vi "xmlparser.vi"(10 "xml_file_content":string="<?xml version=\"1.0\" ?>\n<SC0>\n  <mod0>\n    <ai1>\n      <Cluster>\n        <Name></Name>\n        <NumElts>7</NumElts>\n        <DBL>\n          <Name>max</Name>\n          <Val>10</Val>\n        </DBL>\n        <DBL>\n          <Name>min</Name>\n          <Val>-10</Val>\n        </DBL>\n        <DBL>\n          <Name>factor_a</Name>\n          <Val>22.4</Val>\n        </DBL>\n        <DBL>\n          <Name>factor_b</Name>\n          <Val>0.0</Val>\n        </DBL>\n        <Boolean>\n          <Name>lowpass</Name>\n          <Val>1</Val>\n        </Boolean>\n        <DBL>\n          <Name>lowpassfreq</Name>\n          <Val>60</Val>\n        </DBL>\n        <DBL>\n          <Name>excitation</Name>\n          <Val>0.4</Val>\n        </DBL>\n      </Cluster>\n      <type>VoltageInputExtExc</type>\n      <name>234</name>\n    </ai1>\n    <ai0>\n      <Cluster>\n        <Name></Name>\n        <NumElts>7</NumElts>\n        <DBL>\n          <Name>max</Name>\n          <Val>10</Val>\n        </DBL>\n        <DBL>\n          <Name>min</Name>\n          <Val>-10</Val>\n        </DBL>\n        <DBL>\n          <Name>factor_a</Name>\n          <Val>22.4</Val>\n        </DBL>\n        <DBL>\n          <Name>factor_b</Name>\n          <Val>0.0</Val>\n        </DBL>\n        <Boolean>\n          <Name>lowpass</Name>\n          <Val>1</Val>\n        </Boolean>\n        <DBL>\n          <Name>lowpassfreq</Name>\n          <Val>60</Val>\n        </DBL>\n        <DBL>\n          <Name>excitation</Name>\n          <Val>10</Val>\n        </DBL>\n      </Cluster>\n      <type>VoltageInputIntExc</type>\n      <name>234</name>\n    </ai0>\n  </mod0>\n</SC0>\n", 11 "XPath expression":string) -> (3 "Array 2":string[](array[string]))   [LabVIEW 2011]
uses:
  <vilib>/xml/Close Reference(Node).vi
  <vilib>/xml/NI_XML.lvlib
  Program Files (x86)/National Instruments/LabVIEW 2011/resource/objmgr/DOMUserDefRef.rc
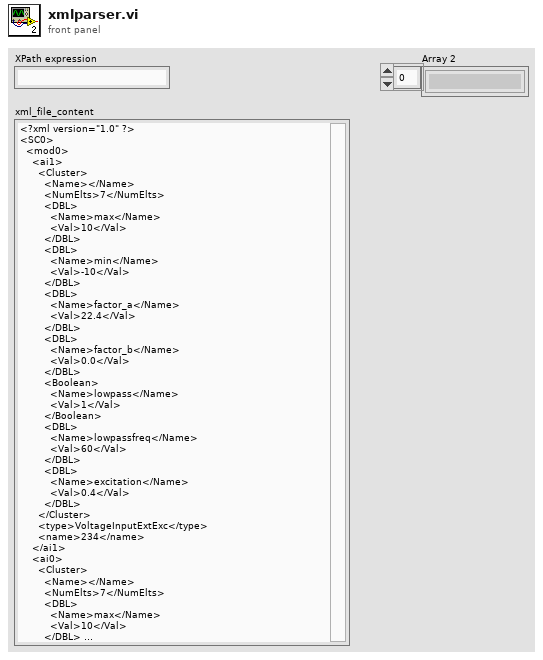
[diagram p1: front panel]
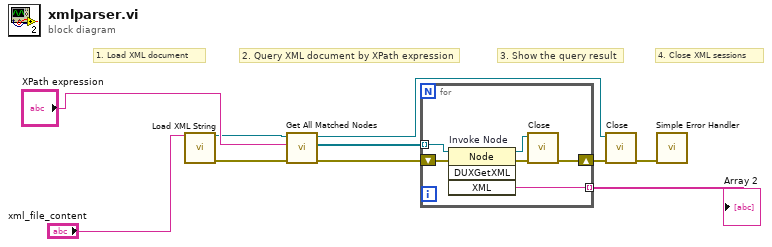
[diagram p0: block diagram]
diagram:
  # "4. Close XML sessions"
  # "3. Show the query result"
  # "2. Query XML document by XPath expression"
  # "1. Load XML document"
  n1 = call <vilib>:"Load XML String.vi"("XML string"="xml_file_content") -> ("DOM document out"=w5:refnum<k20>, "error out"=w4:errorcluster)  [unwired: 1 in, 12 out]
  n2 = call <vilib>:"Get All Matched Nodes.vi"("error in (no error)"=w4, "XPath expression"="XPath expression", "node in"=w5) -> ("error out"=w3:errorcluster, "node result array"=w2:refnum<k20>[], "node out"=w7:refnum<k20>)  [unwired: 6 out]
  n3 = for {
    tunnel: w2 -> [w12] mode=indexing
    shift-right: [w14] -> w6
    shift-left: w3 -> [w13]
    tunnel: [w11] -> w9 mode=indexing
    n4 = invoke on="Invoke Node" class="Node" method="DUXGetXML"(reference=w12, error in=w13) -> (reference out=w15:refnum<k20>, error out=w16:errorcluster, "XML"=w11:string)  [unwired: 2 in, 1 out]
    n5 = call-poly <vilib>:"Close.vi"("error in (no error)"=w16, "node"=w15) -> ("error out"=w14:errorcluster)  [unwired: 7 out]
  }
  "Array 2" <- w9
  n6 = call-poly <vilib>:"Close.vi"("error in (no error)"=w6, "node"=w7) -> ("error out"=w8:errorcluster)  [unwired: 7 out]
  n7 = call <vilib>:"Simple Error Handler.vi"("error in (no error)"=w8) -> ()  [unwired: 1 in, 8 out]
